vi "Topo & GridSpectr_DriftCorrection_zSpec_v16.vi"(6 "Internal use":string, 7 "Grid param":T1 {"height (m)" format="%#_6p"; "width (m)" format="%#_6p"; "center Y (m)" format="%#_6p"; "center X (m)" format="%#_6p"}, 8 "Error in (no error)":errorcluster, 9 "Points Y/Index Y":i32, 10 "Points X/Index X":i32, 11 "Method":enum16{"init", "run", "end"}(ring)=enum."end") -> (0 "Error out":errorcluster)   [LabVIEW 2014]
doc: "Example of a measurement VI to be used in the \"Experiments on a Grid\" tool as external VI.\n\nThis example measure the topography and spectroscopy data. The spectroscopy measurements are taken on a subgrid. The data are saved to a sxm and a binary file.\n\n- Nanonis Programming Interface -"
uses:
  <userlib>/Nanonis Prog Interface V5/Scan/Grid/GridPatternGet.vi
  <userlib>/Nanonis Prog Interface V5/Scan/Grid/LinePatternGet.vi
  <userlib>/Nanonis Prog Interface V5/Nanonis Prog Interface.lvlib
panel:
  in  "autoStop":bool
  in  "trigger 2 >Hz":sgl format="%#_6p"
  in  "trigger1 < Hz":sgl format="%#_6p"
  out "zFile":refnum<file>
  out "last z adjustment":sgl format="%#_6p"
  in  "during Spec Bias (V)":sgl format="%#_5p"
  in  "type":u16(ring)=1 items=["Line", "Grid"]
  in  "readjust setpoint every":i32=4
  in  "Correct Drift":bool=TRUE
  in  "Email when finished":string="cornelius.krull@monash.edu"
  in  "STS z offset":dbl format="%#_6p"
  out "ETA":timestamp
  out "remaining":dbl format="%<%H:%M:%S>t"
  out "Progress":u8(slide) scale=0.0..100.0 scale format="%#.1g"
  out "total Points":i32
  in  "preSTS delay [ms]":u32=500
  in  "ref Bias":dbl=0.02 format="%#_6p"
  in  "Imaging Bias":dbl=0.02 format="%#_6p"
  in  "max applied Drift Correction":i32=20 min=1 max=100 step=1 format="%.0p"
  in  "Correlate":u16(ring) items=["first Frame", "successive Frames"]
  out "Topo Images taken":i32=14
  in  "Increment":i32=40
  in  "Threshold":i32=2 min=1 step=1
  in  "tip Speed (m/s)":sgl=2e-09 format="%.2p"
  out "X drift":i32
  out "Y drift":i32
  out "Last Drift detected":i32=40
  in  "MaxImagesBack":i32=40
  in  "Channel index (0-23)":u8(ring) items=["Current"=0, "Z (m)"=14]
  in  "File name":string="symmetric_node"
  in  "ref Current":dbl=5e-12 format="%#_6p"
  in  "Imaging Current":dbl=5e-12 format="%#_6p"
  in  "zdrift \nDuration (s)":dbl
  in  "Correct z drift":bool
  out "Status":string="finishing"
  in  "Drift correction Pixels":i32=256 caption="Topo Pixels"
  out "Y Offset":dbl format="%#_6p"
  out "X Offset":dbl format="%#_6p"
  out "Points taken":dbl=14.0
  in  "Drift Correction every":i32=40
  # "z Spectroscopy"
  # "GRID points"
  # "Increase this if no Drift was detected for \na certain number of images"
  # "%"
  # "time (HH:MM:SS)"
  # "images back"
  # "% of image size"
  # "RUN smart tilt before starting the GRID\nImg Angle = 0\nmove tip to reference point for tip height"
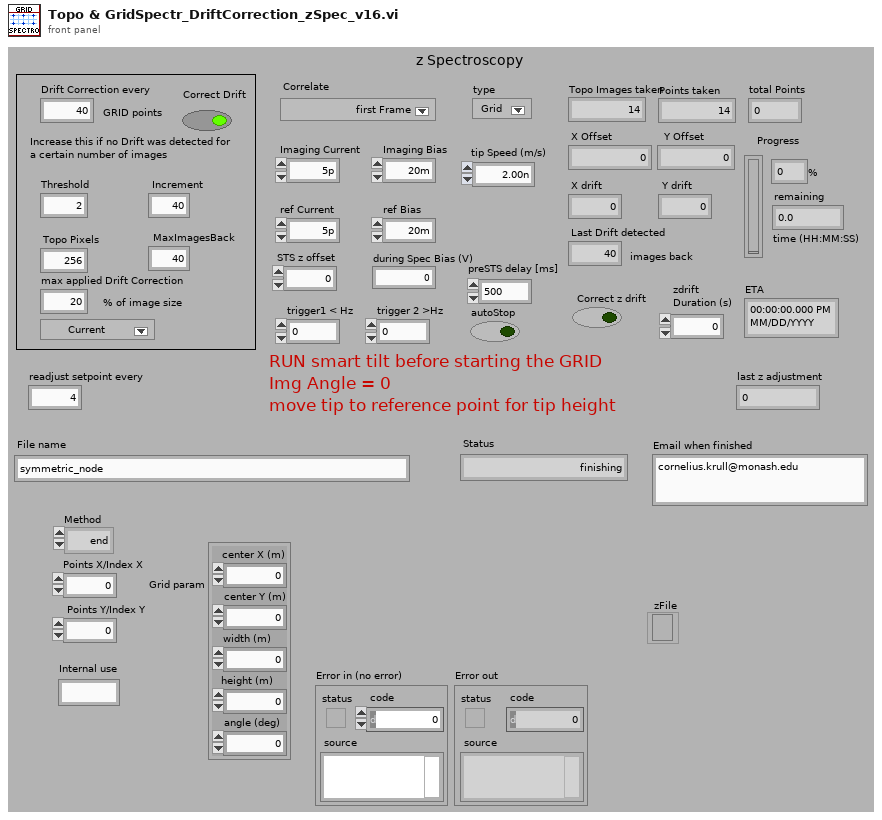
[diagram p1: front panel]
types:
  T1 = cluster{"center X (m)":sgl, "center Y (m)":sgl, "width (m)":sgl, "height (m)":sgl, "angle (deg)":sgl}
  T2 = enum16{"open", "replace", "create", "open or create", "replace or create", "replace or create with confirmation"}
  T3 = cluster{"Z averaging time (s)":sgl, "Z offset (m)":sgl, "Initial settling time (s)":sgl}
  T4 = cluster{"Drift correction Pixels":i32, "Imaging Current":dbl, "STS Current":dbl, "MaxImagesBack":i32, "tip Speed (m/s)":sgl, "Threshold":i32, "Increment":i32, "Correlate":u16, "max applied Drift Correction":i32, "Imaging Bias":dbl, "Move Current":dbl, "Move Bias":dbl, "STS Bias":dbl, "preSTS delay [ms]":u32, "STS z offset":dbl, "Correct Drift":bool, "Lockin ON/OFF":bool}
  T5 = cluster{"center X":sgl, "center Y":sgl, "angle":sgl, "width":sgl, "height":sgl, "# pixels":i32, "# lines":i32}
  T6 = cluster{"Name":string, "Calibration":sgl, "Offset":sgl, "Channel index":i32}[]
  T7 = cluster{"up/down":bool, "time/line":sgl, "start time":timestamp, "end time":timestamp}
  T8 = cluster{"Points X/Index X":i32, "Points Y/Index Y":i32}
  T9 = cluster{"Z averaging time (s)":sgl, "Initial settling time (s)":sgl}
  T10 = cluster{"Max. slew rate (m/s)":sgl, "Settling time (s)":sgl, "Integration time (s)":sgl}
  T11 = cluster{"End settling time (s)":sgl, "Z control time (s)":sgl}
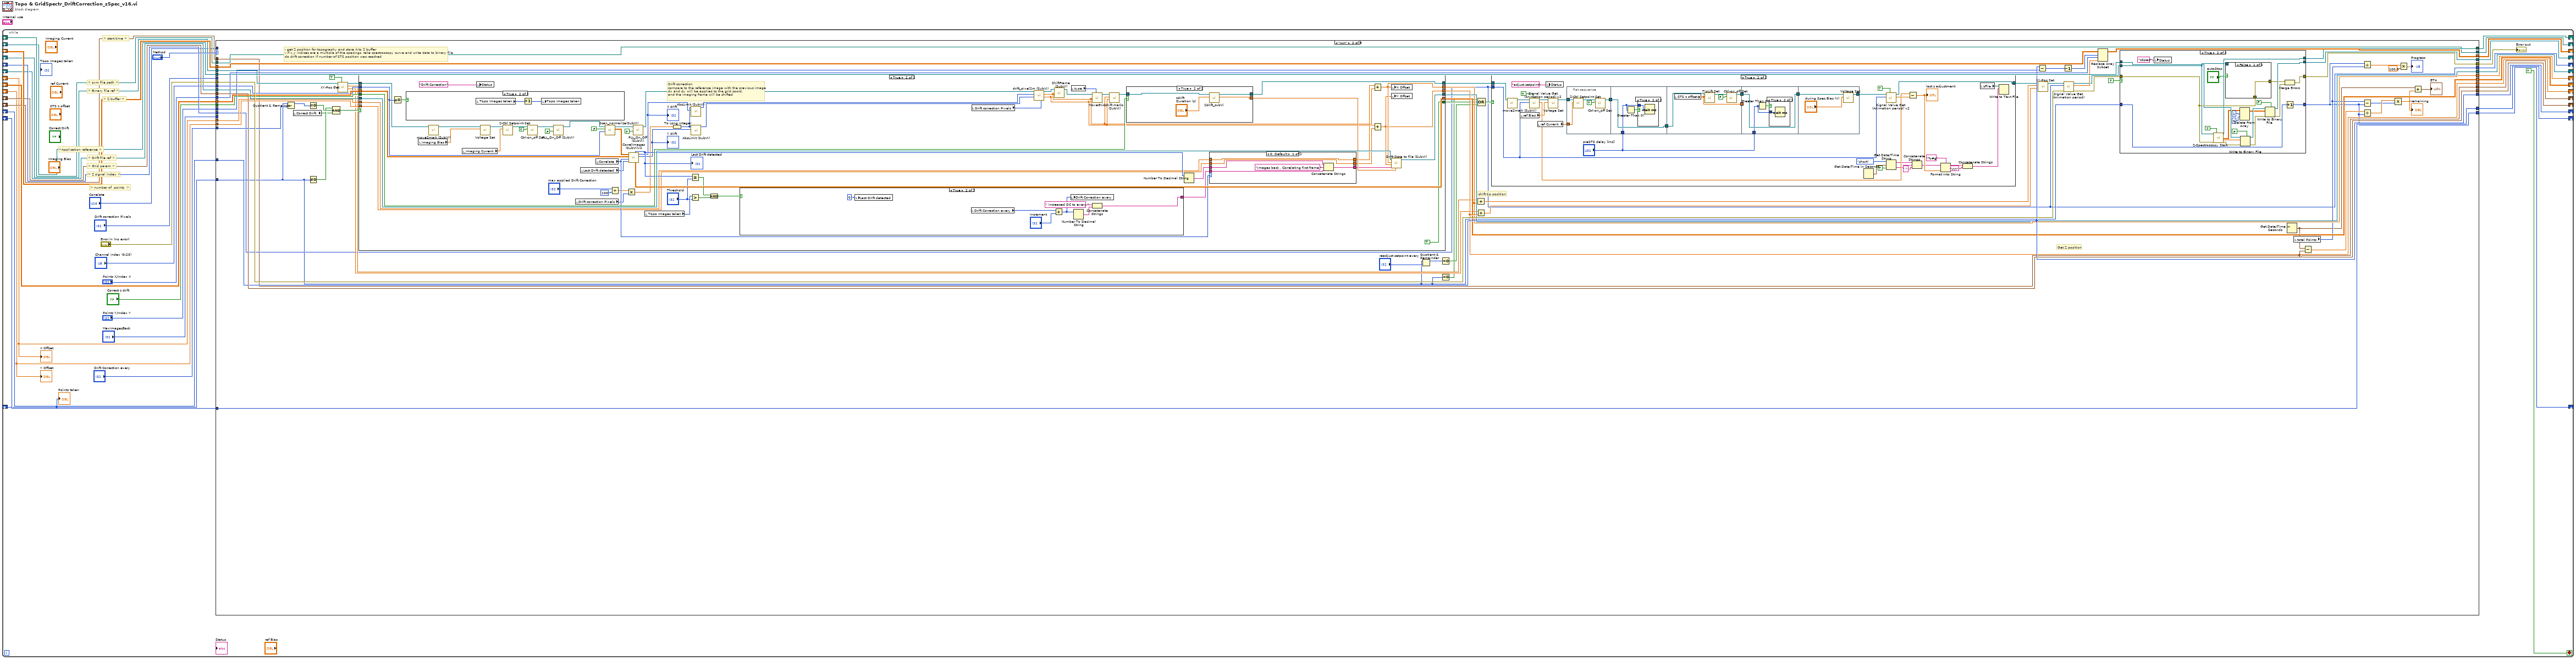
[diagram p0: block diagram]
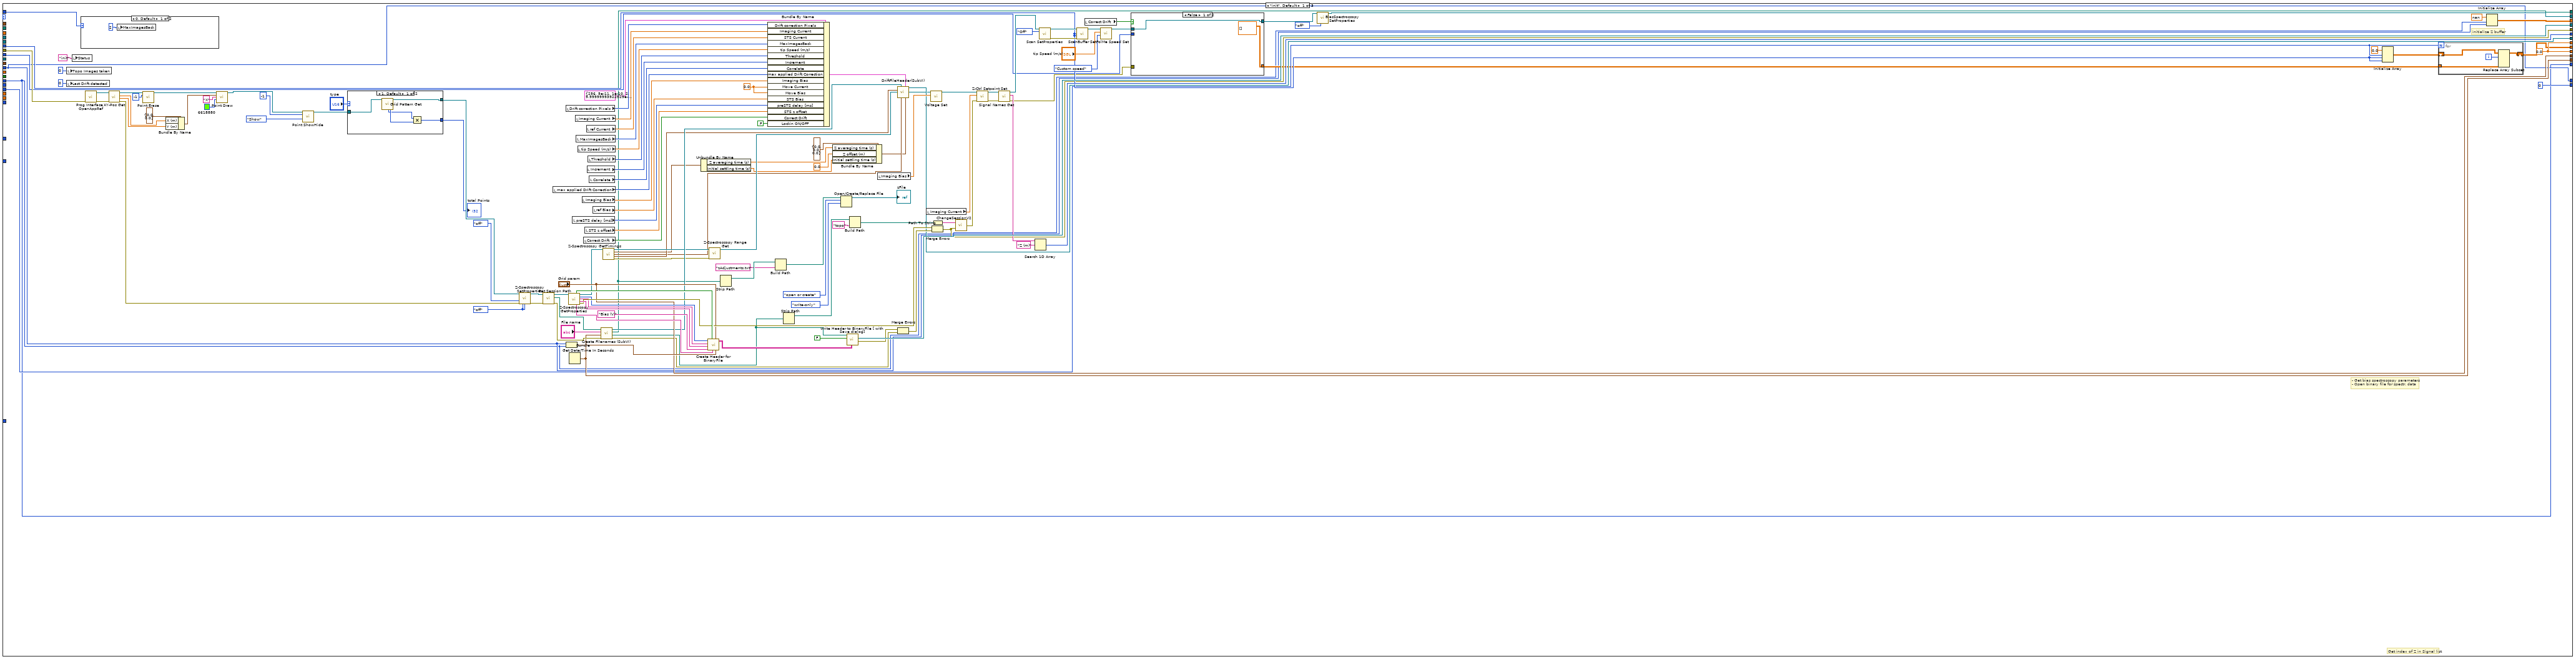
[diagram p2: hidden frame]
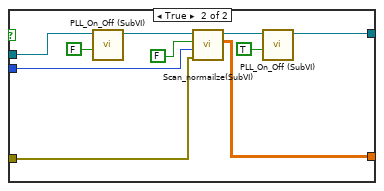
[diagram p3: hidden frame]
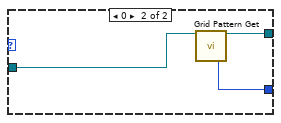
[diagram p4: hidden frame]
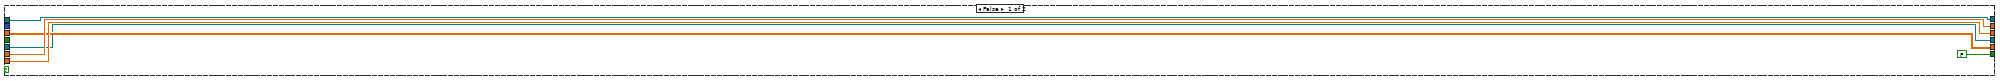
[diagram p9: hidden frame]
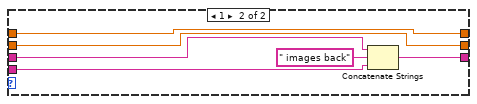
[diagram p10: hidden frame]
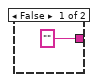
[diagram p12: hidden frame]
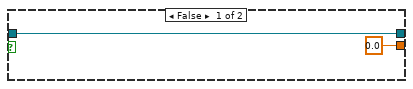
[diagram p13: hidden frame]
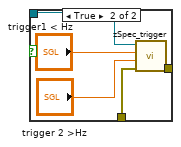
[diagram p15: hidden frame]
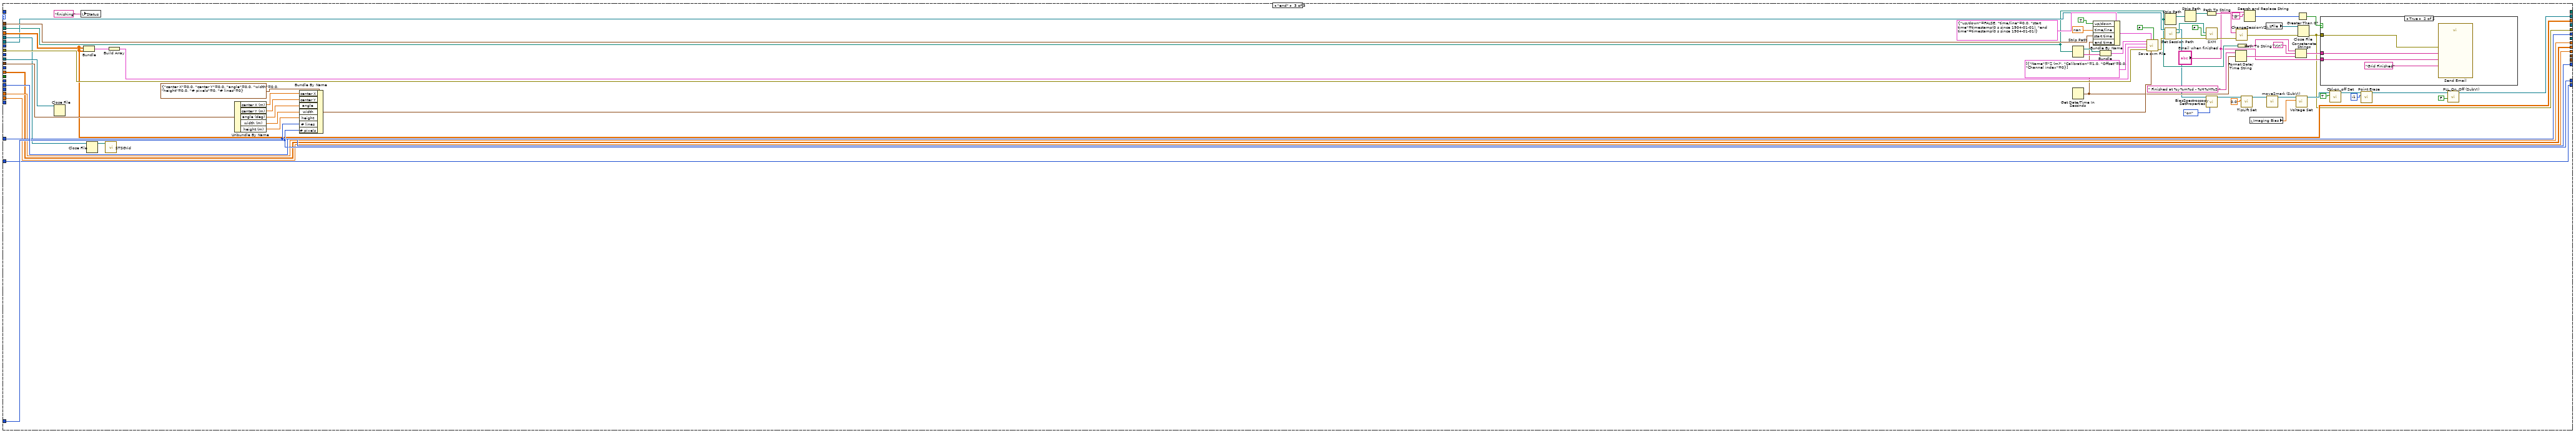
[diagram p16: hidden frame]
diagram:
  n1 = while {
    shift-right: [w21] -> _
    shift-left: _ -> [w38]
    shift-right: [w33] -> _
    shift-left: _ -> [w32]
    shift-right: [w30] -> _
    shift-left: _ -> [w31]
    shift-right: [w29] -> _
    shift-left: _ -> [w28]
    shift-right: [w27] -> _
    shift-left: _ -> [w26]
    shift-right: [w25] -> _
    shift-left: _ -> [w24]
    shift-right: [w23] -> _
    shift-left: _ -> [w22]
    shift-right: [w20] -> _
    shift-left: _ -> [w19]
    shift-right: [w18] -> _
    shift-left: _ -> [w17]
    shift-right: [w16] -> _
    shift-left: _ -> [w9]
    shift-right: [w15] -> _
    shift-left: _ -> [w8]
    shift-right: [w14] -> _
    shift-left: _ -> [w11]
    shift-right: [w13] -> _
    shift-left: _ -> [w10]
    shift-right: [w6] -> _
    shift-left: _ -> [w5]
    stop <- TRUE stop-if-true
    # "> Drift file ref >"
    # "> number of  points  >"
    # "> Grid param >"
    # "> start time >"
    # ">Application reference >"
    # "> Z signal index >"
    # "> Binary file ref >"
    # "> Z buffer >"
    # "> sxm file path >"
    n2 = case shown="\"run\"" "Method" {
      tunnel: [w49 w259 _] -> w21
      tunnel: w38 -> [_ w259 w470]
      tunnel: "Error in (no error)" -> [w143 w252 w500]
      tunnel: [w123 w258 w447] -> w36
      tunnel: "Points X/Index X" -> [w42 w253 _]
      tunnel: "Points Y/Index Y" -> [w41 w246 _]
      tunnel: [w169 w256 w489] -> w33
      tunnel: w32 -> [_ w257 w489]
      tunnel: w31 -> [_ w255 w482]
      tunnel: [w161 w254 _] -> w30
      tunnel: [w159 w196 w512] -> w29
      tunnel: w28 -> [_ w196 w512]
      tunnel: [w108 w239 w445] -> w27
      tunnel: w26 -> [_ w223 w475]
      tunnel: ["Grid param" w249 _] -> w25
      tunnel: w24 -> [_ w249 w499]
      tunnel: [w141 w214 _] -> w23
      tunnel: w22 -> [_ w214 w507]
      tunnel: [w41 w247 w490] -> w20
      tunnel: w19 -> [_ w247 w490]
      tunnel: [w42 w248 w491] -> w18
      tunnel: w17 -> [_ w248 w491]
      tunnel: [w152 w229 w488] -> w16
      tunnel: [w152 w234 w486] -> w15
      tunnel: [w137 w228 w483] -> w14
      tunnel: [0 w212 w487] -> w13
      tunnel: w10 -> [_ w198 w487]
      tunnel: "Drift Correction every" -> [_ w242 _]
      tunnel: w11 -> [_ w233 w483]
      tunnel: w9 -> [_ w240 w488]
      tunnel: w8 -> [_ w226 w486]
      tunnel: "Drift correction Pixels" -> [w136 _ _]
      tunnel: [w104 w231 _] -> w6
      tunnel: w5 -> [_ w232 w484]
      tunnel: "Correct z drift" -> [_ w230 _]
      tunnel: "Channel index (0-23)" -> [w86 w227 _]
      tunnel: "MaxImagesBack" -> [w135 _ _]
      tunnel: "Correlate" -> [w116 _ _]
      frame "init", Default {
        w51 = 0.0 ("Move Current")
        w106 = enum16{"no change", "on", "off"}."off" ("Save dialog")
        w152 = 0.0
        # "- Get bias spectroscopy parameters\n- Open binary file for spectr. data"
        # "initialize Z buffer"
        # "Get index of Z in Signal list"
        n3 = local write "Topo Images taken"(0 ("Images taken")) -> ()
        n4 = local write "Last Drift detected"(0 ("Last Drift detected")) -> ()
        n5 = local write "Status"("init" ("Status")) -> ()
        n6 = case shown="0, Default" w116 {
          frame 0, Default {
            n7 = local write "MaxImagesBack"(2 ("StepsBack")) -> ()
          }
          frame 1 {
          }
        }
        n8 = call <userlib>:"Prog Interface - OpenAppRef.vi"("Error in (no error)"=w143) -> ("Error out"=w81:errorcluster, "Application reference"=w83:refnum<vi>)  [unwired: 5 in]
        n9 = call <userlib>:"XY-Pos Get.vi"("error in (no error)"=w81, "Application ref in"=w83) -> ("error out"=w82:errorcluster, "Y (m)"=w75:sgl, "X (m)"=w76:sgl, "Application ref out"=w57:refnum<vi>)  [unwired: 5 in]
        n10 = call <userlib>:"Point Erase.vi"("Application ref in"=w57, "Point index (-1=All points)"=-1) -> ("Application ref out"=w56:refnum<vi>)  [unwired: 12 in, 1 out]
        n11 = Bundle By Name(cluster=cluster{"X (m)":sgl, "Y (m)":sgl} {"X (m)"=0.0, "Y (m)"=0.0} ("Point Coordinates"), "X (m)"=w76, "Y (m)"=w75) -> (w77:cluster{"X (m)":sgl, "Y (m)":sgl})
        n12 = call <userlib>:"Point Draw.vi"("Application ref in"=w56, "Point Coordinates"=w77, "Text"="X", "Color"=u32 6618880) -> ("Application ref out"=w61:refnum<vi>)  [unwired: 10 in, 1 out]
        n13 = call <userlib>:"Point ShowHide.vi"("Application ref in"=w61, "Point index (-1=All points)"=-1, "Show/Hide"=enum16{"Show", "Hide"}."Show") -> ("Application ref out"=w60:refnum<vi>)  [unwired: 11 in, 1 out]
        n14 = case shown="1, Default" "type" {
          tunnel: [w186 w189] -> w110
          tunnel: [w183 w187] -> w109
          tunnel: w60 -> [w182 w188]
          frame 1, Default {
            n15 = call-poly <userlib>:"Grid Pattern Get.vi"("Application ref in"=w182) -> ("Points Y"=w184:i32, "Points X"=w185:i32, "Application ref out"=w186:refnum<vi>)  [unwired: 10 in, 6 out]
            n16 = Multiply(x=w184, y=w185) -> (x*y=w183:i32)
          }
          frame 0 {
            n17 = call-poly <userlib>:"Grid Pattern Get.vi"("Application ref in"=w188) -> ("Points"=w187:i32, "Application ref out"=w189:refnum<vi>)  [unwired: 12 in, 5 out]
          }
        }
        "total Points" <- w109
        n18 = call <userlib>:"Z-Spectroscopy SetProperties.vi"("Application ref in"=w110, "Autosave"=enum16{"no change", "on", "off"}."off" ("Autosave (no change)"), "error in (no error)"=w82, "Save dialog"=w106, "Save all sweeps (no change)"=w106) -> ("Application ref out"=w119:refnum<vi>, "error out"=w118:errorcluster)  [unwired: 9 in]
        n19 = call <userlib>:"Get Session Path.vi"("error in (no error)"=w118, "Application ref in"=w119) -> ("error out"=w142:errorcluster, "Session path"=w129:path, "Application ref out"=w120:refnum<vi>)  [unwired: 7 in]
        n20 = local read "max applied Drift Correction"() -> (w92:i32)
        n21 = local read "Drift correction Pixels"() -> (w100:i32)
        n22 = Bundle("Points X/Index X"=w42, "Points Y/Index Y"=w41) -> (w164:T8)  [unwired: 1 in]
        n23 = call <userlib>:"Z-Spectroscopy GetProperties.vi"("Application ref in"=w120) -> ("Backward sweep"=w165:bool, "Application ref out"=w72:refnum<vi>, "Number of points"=w156:i32, "Channels"=w155:string[], "Parameters"=w163:string[], "Fixed parameters"=w158:string[], "error out"=w162:errorcluster)  [unwired: 7 in, 1 out]
        n24 = Get Date/Time In Seconds() -> (seconds since 1Jan1904=w141:timestamp)
        n25 = local read "preSTS delay [ms]"() -> (w89:u32)
        n26 = local read "Imaging Current"() -> (w99:dbl)
        n27 = local read "MaxImagesBack"() -> (w96:i32)
        n28 = local read "tip Speed (m/s)"() -> (w97:sgl)
        n29 = local read "Imaging Bias"() -> (w91:dbl)
        n30 = local read "Correct Drift"() -> (w87:bool)
        n31 = local read "STS z offset"() -> (w88:dbl)
        n32 = local read "ref Current"() -> (w98:dbl)
        n33 = local read "Increment"() -> (w94:i32)
        n34 = local read "Threshold"() -> (w95:i32)
        n35 = local read "Correlate"() -> (w93:u16)
        n36 = local read "ref Bias"() -> (w90:dbl)
        n37 = call "Create Filenames (SubVI).vi"("error in (no error)"=w142, "seconds since 1Jan1904"=w141, "File name"="File name", "Session path"=w129) -> ("error out"=w132:errorcluster, "binFilePath"=w125:path, "topoFilePath"=w49:path, "Drift File out"=w105:refnum<file>)  [unwired: 4 in]
        n38 = call <userlib>:"Z-Spectroscopy GetTimings.vi"("Application ref in"=w72) -> ("Application ref out"=w73:refnum<vi>, "Initialization"=w68:T9, "Sweep Timing"=w69:T10, "End of Sweep"=w70:T11, "Error out"=w74:errorcluster)  [unwired: 10 in]
        n39 = Unbundle By Name(w68) -> ("Z averaging time (s)"=w65:sgl, "Initial settling time (s)"=w64:sgl)
        n40 = call <userlib>:"Create Header for BinaryFile.vi"("Grid points"=w164, "Grid param"="Grid param", "Fixed parameters"=w158, "Backward sweep"=w165, "Sweep signal"="Bias (V)" ("Sweep Signal"), "Parameters"=w163, "Channels"=w155, "Points per sweep"=w156) -> ("Header (fixed attributes)"=w167:string[][])  [unwired: 3 in]
        n41 = call <userlib>:"Z-Spectroscopy Range Get.vi"("error in (no error)"=w74, "Application ref in"=w73) -> ("Application ref out"=w71:refnum<vi>)  [unwired: 5 in, 3 out]
        n42 = Strip Path(path=w49) -> (stripped path=w48:path)  [unwired: 1 out]
        n43 = Bundle By Name(cluster=T4 {"Drift correction Pixels"=256, "Imaging Current"=5e-11, "STS Current"=1e-10, "MaxImagesBack"=2, "tip Speed (m/s)"=1e-08, "Threshold"=2, "Increment"=64, "Correlate"=0, "max applied Drift Correction"=20, "Imaging Bias"=-0.02, "Move Current"=1.5e-11, "Move Bias"=-0.02, "STS Bias"=0.1, "preSTS delay [ms]"=1000, "STS z offset"=-1.7e-10, "Correct Drift"=TRUE, "Lockin ON/OFF"=TRUE} ("Drift Correction"), "Drift correction Pixels"=w100, "Imaging Current"=w99, "STS Current"=w98, "MaxImagesBack"=w96, "tip Speed (m/s)"=w97, "Threshold"=w95, "Increment"=w94, "Correlate"=w93, "max applied Drift Correction"=w92, "Imaging Bias"=w91, "Move Current"=w51, "Move Bias"=w51, "STS Bias"=w90, "preSTS delay [ms]"=w89, "STS z offset"=w88, "Correct Drift"=w87, "Lockin ON/OFF"=FALSE) -> (w102:T4)
        n44 = Build Path(base path=w48, name or relative path="zAdjustments.txt") -> (appended path=w46:path)
        n45 = Strip Path(path=w125) -> (stripped path=w128:path)  [unwired: 1 out]
        n46 = Bundle By Name(cluster=T3 {"Z averaging time (s)"=0.0, "Z offset (m)"=0.0, "Initial settling time (s)"=0.0} ("Initialization"), "Z averaging time (s)"=w65, "Z offset (m)"=sgl 0.0, "Initial settling time (s)"=w64) -> (w66:T3)
        n47 = Open/Create/Replace File(file path (use dialog)=w46, operation (0:open)=T2."open or create", access (0:read/write)=enum16{"read/write", "read-only", "write-only"}."write-only") -> (refnum out=→"zFile":refnum<file>)  [unwired: 3 in, 2 out]
        n48 = call <userlib>:"Write Header to BinaryFile [ with Save dialog].vi"("Fixed Attributes"=w167, "Show Dialog? (T)"=FALSE, "Filename"=w125) -> ("Error out"=w133:errorcluster, "File ref"=w161:refnum<file>)  [unwired: 5 in, 2 out]
        n49 = Build Path(base path=w128, name or relative path="topo") -> (appended path=w126:path)
        n50 = local read "Imaging Bias"() -> (w112:dbl)
        n51 = call "DriftFileHeader(SubVI).vi"("Byte Stream File in"=w105, "Drift Correction"=w102, "End of Sweep"=w70, "Application ref in"=w71, "Sweep Timing"=w69, "Initialization"=w66) -> ("Byte Stream File out"=w104:refnum<file>, "Application ref out"=w103:refnum<vi>)  [unwired: 8 in]
        n52 = Merge Errors(w133, w132) -> (w134:errorcluster)
        n53 = local read "Imaging Current"() -> (w111:dbl)
        n54 = call <userlib>:"Voltage Set.vi"("Bias (V)"=w112, "Application ref in"=w103) -> ("Application ref out"=w113:refnum<vi>)  [unwired: 8 in, 1 out]
        n55 = Path To String(path=w126) -> (string=w124:string)
        n56 = Merge Errors(w162, w134) -> (w123:errorcluster)
        n57 = call "ChangeSessionV2.vi"("error in (no error)"=w123, "Session"=w124) -> ("error out"=w122:errorcluster)
        n58 = call <userlib>:"Z-Ctrl Setpoint Set.vi"("error in (no error)"=w122, "Z Controller setpoint"=w111, "Application ref in"=w113) -> ("error out"=w144:errorcluster, "Application ref out"=w145:refnum<vi>)  [unwired: 7 in]
        n59 = call <userlib>:"Signal Names Get.vi"("error in (no error)"=w144, "Application ref in"=w145) -> ("error out"=w85:errorcluster, "Signals Names"=w157:string[], "Application ref out"=w148:refnum<vi>)  [unwired: 5 in]
        n60 = Search 1D Array(1D array=w157, element="Z (m)") -> (index of element=w159:i32)  [unwired: 1 in]
        n61 = call <userlib>:"Scan SetProperties.vi"("Application ref in"=w148, "Continuous scan"=enum16{"No change", "On", "Off"}."Off") -> ("Application ref out"=w150:refnum<vi>, "Error out"=w149:errorcluster)  [unwired: 12 in]
        n62 = call <userlib>:"ScanBuffer Set.vi"("Application ref in"=w150, "Pixels"=w136, "Lines"=w136, "error in (no error)"=w149) -> ("Application ref out"=w114:refnum<vi>)  [unwired: 10 in, 1 out]
        n63 = local read "Correct Drift"() -> (w52:bool)
        n64 = call <userlib>:"FolMe Speed Set.vi"("Speed Setting (Custom)"=enum32{"Scan speed", "Custom speed"}."Custom speed", "Speed (m/s)"="tip Speed (m/s)", "Application ref in"=w114) -> ("Application ref out"=w54:refnum<vi>)  [unwired: 5 in, 1 out]
        n65 = case shown="False" w52 {
          tunnel: w86 -> [_ w181]
          tunnel: w85 -> [_ w180]
          tunnel: [dbl[][] [] ("Array") w179] -> w84
          tunnel: w54 -> [w171 w177]
          tunnel: [w171 w172] -> w50
          frame False {
          }
          frame True {
            n66 = call "PLL_On_Off (SubVI).vi"("Output ON/OFF (F=OFF)"=FALSE, "Application in"=w177) -> ("Application out"=w176:refnum<vi>)  [unwired: 8 in, 1 out]
            n67 = call "Scan_normailze(SubVI).vi"("error in (no error)"=w180, "Channel index (0-23)"=w181, "Normalization"=FALSE ("Boolean"), "Application in"=w176) -> ("Array"=w179:dbl[][], "Application out"=w173:refnum<vi>)  [unwired: 5 in, 1 out]
            n68 = call "PLL_On_Off (SubVI).vi"("Output ON/OFF (F=OFF)"=TRUE, "Application in"=w173) -> ("Application out"=w172:refnum<vi>)  [unwired: 8 in, 1 out]
          }
        }
        n69 = call <userlib>:"BiasSpectroscopy SetProperties.vi"("Application ref in"=w50, "Z-Controller hold (no change)"=enum16{"no change", "on", "off"}."off") -> ("Application ref out"=w108:refnum<vi>)  [unwired: 12 in, 1 out]
        n70 = Initialize Array(0.0 ("element"), w135, w136, w136) -> (w138:dbl[][][])
        n71 = for {
          N: w135 -> [_]
          tunnel: w84 -> [w193]
          shift-right: [w192] -> w137
          shift-left: w138 -> [w194]
          i -> [w191]
          n72 = Replace Array Subset(array=w194, new element=w193, index (dim 0)=w191) -> (w192:dbl[][][])  [unwired: 2 in]
        }
        n73 = Initialize Array(sgl nan ("element"), w41, w42) -> (w169:sgl[][])
      }
      frame "run" {
        # "shift tip position"
        # "Get Z position"
        # "- get Z position for topography and store it to Z buffer\n- if x,y indices are a multiple of the spacings, take spectroscopy curve and write data to binary file\ndo drift correction if number of STS position was reached"
        n74 = Quotient & Remainder(x=w198, y=w242) -> (x-y*floor(x/y)=w243:i32)  [unwired: 1 out]
        n75 = local read "Correct Drift"() -> (w206:bool)
        n76 = Equal To 0?(x=w243) -> (x = 0?=w241:bool)
        n77 = Not Equal To 0?(x=w198) -> (x != 0?=w224:bool)
        n78 = Compound Arithmetic op=AND(w224, w241, w206) -> (w225:bool)
        n79 = call <userlib>:"XY-Pos Get.vi"("Wait for newest data (F=False)"=TRUE, "Application ref in"=w223) -> ("Y (m)"=w219:sgl, "X (m)"=w220:sgl, "Application ref out"=w222:refnum<vi>)  [unwired: 5 in, 1 out]
        n80 = case shown="True" w225 {
          tunnel: w222 -> [w320 w332]
          tunnel: [w320 w377] -> w203
          tunnel: w233 -> [w317 w373]
          tunnel: [w319 w375] -> w229
          tunnel: [w318 w374] -> w234
          tunnel: w240 -> [w319 w356]
          tunnel: w226 -> [w318 w354]
          tunnel: [w317 w369] -> w228
          tunnel: w232 -> [w316 w380]
          tunnel: [w316 w379] -> w231
          tunnel: w230 -> [_ w376]
          tunnel: w227 -> [_ w360]
          tunnel: [FALSE TRUE] -> w200
          frame False {
          }
          frame True {
            # "Drift correction \ncompare to the reference image with the previous image \ndx and dy will be applied to the grid coord, \nand the imaging frame will be shifted"
            n81 = Greater Or Equal To 0?(x=w360) -> (x >= 0?=w359:bool)
            n82 = case shown="True" w359 {
              frame False {
              }
              frame True {
                n83 = local read "Topo Images taken"() -> (w395:i32)
                n84 = Increment(x=w395) -> (x+1=w394:i32)
                n85 = local write "Topo Images taken"(w394) -> ()
              }
            }
            n86 = local read "Imaging Bias"() -> (w339:dbl)
            n87 = call "move2mark (SubVI).vi"("Application in"=w332) -> ("Application out"=w331:refnum<vi>)  [unwired: 10 in]
            n88 = local read "Imaging Current"() -> (w338:dbl)
            n89 = local write "Status"("Drift Correction" ("Status")) -> ()
            n90 = call <userlib>:"Voltage Set.vi"("Bias (V)"=w339, "Application ref in"=w331) -> ("Application ref out"=w340:refnum<vi>)  [unwired: 8 in, 1 out]
            n91 = call <userlib>:"Z-Ctrl Setpoint Set.vi"("Z Controller setpoint"=w338, "Application ref in"=w340) -> ("Application ref out"=w330:refnum<vi>)  [unwired: 8 in, 1 out]
            n92 = call <userlib>:"Ctrl-on_off Set.vi"("Z Controller ON/OFF"=TRUE, "Application ref in"=w330) -> ("Application ref out"=w328:refnum<vi>)  [unwired: 8 in, 1 out]
            n93 = call "PLL_On_Off (SubVI).vi"("Output ON/OFF (F=OFF)"=FALSE, "Application in"=w328) -> ("Application out"=w327:refnum<vi>)  [unwired: 8 in, 1 out]
            n94 = local read "Drift correction Pixels"() -> (w348:i32)
            n95 = local read "Last Drift detected"() -> (w351:i32)
            n96 = local read "Correlate"() -> (w357:u16)
            n97 = call "Scan_normailze(SubVI).vi"("Channel index (0-23)"=w360, "Normalization"=FALSE ("Boolean"), "Application in"=w327) -> ("Array"=w370:dbl[][], "Application out"=w325:refnum<vi>)  [unwired: 6 in, 1 out]
            n98 = Divide(x="max applied Drift Correction", y=100) -> (x/y=w347:dbl)
            n99 = Multiply(x=w347, y=w348) -> (x*y=w349:dbl)
            n100 = call "CorrelImages (SubVI)v2.vi"("last drift detected"=w351, "Correlate"=w357, "Ref Array"=w373, "New Image"=w370) -> ("Y drift"=w345:i32, "X drift"=w342:i32, "Ref Array out"=w369:dbl[][][], "Queue Steps"=w358:i32)  [unwired: 4 in]
            "X drift" <- w342
            "Y drift" <- w345
            "Last Drift detected" <- w358
            n101 = call "PLL_On_Off (SubVI).vi"("Output ON/OFF (F=OFF)"=TRUE, "Application in"=w325) -> ("Application out"=w322:refnum<vi>)  [unwired: 8 in, 1 out]
            n102 = local read "Topo Images taken"() -> (w362:i32)
            n103 = To Long Integer(number=w349) -> (32bit integer=w341:i32)
            n104 = Greater Or Equal?(x=w358, y="Threshold") -> (x >= y?=w364:bool)
            n105 = Greater?(x=w362, y="Threshold") -> (0:w361:bool)
            n106 = call "AbsLimit (SubVI).vi"("in"=w342, "Abslimt"=w341) -> ("Numeric out"=w344:i32)  [unwired: 9 in]
            n107 = call "AbsLimit (SubVI).vi"("in"=w345, "Abslimt"=w341) -> ("Numeric out"=w343:i32)  [unwired: 9 in]
            n108 = And(x=w364, y=w361) -> (x .and. y?=w363:bool)
            n109 = case shown="True" w363 {
              tunnel: ["" w399] -> w365
              frame False {
              }
              frame True {
                n110 = local write "Last Drift detected"(0 ("Last Drift detected")) -> ()
                n111 = local read "Drift Correction every"() -> (w398:i32)
                n112 = Add(x=w398, y="Increment") -> (x+y=w402:i32)
                n113 = local write "Drift Correction every"(w402) -> ()
                n114 = Number To Decimal String(number=w402) -> (decimal integer string=w401:string)  [unwired: 1 in]
                n115 = Concatenate Strings(" Increased DC to every " ("string"), w401) -> (w399:string)
              }
            }
            n116 = local read "Drift correction Pixels"() -> (w367:i32)
            n117 = call "drift_pixel2m (SubVI).vi"("Application in"=w322, "X drift"=w344, "Y drift"=w343, "Drift correction Pixels"=w367) -> ("Application out"=w366:refnum<vi>, "x drift"=w336:sgl, "y drift"=w335:sgl)  [unwired: 2 in, 1 out]
            n118 = call "ShiftFrame (SubVI).vi"("Y shift"=w335, "X shift"=w336, "Application in"=w366) -> ("Application out"=w368:refnum<vi>)  [unwired: 8 in]
            n119 = local read "type"() -> (w321:u16)
            n120 = call "MoveGrid.vi"("type"=w321, "y"=w335, "x"=w336, "Application ref in"=w368) -> ("Application ref out"=w334:refnum<vi>)  [unwired: 6 in, 1 out]
            n121 = call "shift marks (SubVI).vi"("y"=w335, "x"=w336, "Application in"=w334) -> ("Application out"=w333:refnum<vi>)  [unwired: 7 in, 1 out]
            n122 = case shown="True" w376 {
              tunnel: [0.0 ("z drift") w409] -> w378
              tunnel: w333 -> [w404 w408]
              tunnel: [w404 w407] -> w377
              frame False {
              }
              frame True {
                n123 = call "Zdrift_subVi.vi"("Duration"="zdrift \nDuration (s)", "Application in"=w408) -> ("z drift"=w409:dbl, "Application out"=w407:refnum<vi>)  [unwired: 7 in, 1 out]
              }
            }
            n124 = Number To Decimal String(number=w358) -> (decimal integer string=w372:string)  [unwired: 1 in]
            n125 = case shown="0, Default" w357 {
              tunnel: w372 -> [w382 w393]
              tunnel: [w387 w392] -> w371
              tunnel: w365 -> [w385 w390]
              tunnel: w356 -> [w383 w389]
              tunnel: [w383 w389] -> w355
              tunnel: w354 -> [w384 w388]
              tunnel: [w384 w388] -> w353
              frame 0, Default {
                n126 = Concatenate Strings(w382, "images back , Correlating first frame " ("string"), w385) -> (w387:string)
              }
              frame 1 {
                n127 = Concatenate Strings(w393, " images back" ("string"), w390) -> (w392:string)
              }
            }
            n128 = Add(x=w355, y=w336) -> (x+y=w375:dbl)
            n129 = Add(x=w335, y=w353) -> (x+y=w374:dbl)
            n130 = local write "X Offset"(w375) -> ()
            n131 = local write "Y Offset"(w374) -> ()
            n132 = call "Drift Data to file (SubVI).vi"("z drift"=w378, "Comment"=w371, "y Drift"=w374, "X drift"=w375, "Byte Stream File in"=w380) -> ("Byte Stream File out"=w379:refnum<file>)  [unwired: 6 in]
          }
        }
        n133 = Quotient & Remainder(x=w198, y="readjust setpoint every") -> (x-y*floor(x/y)=w199:i32)  [unwired: 1 out]
        n134 = Equal To 0?(x=w199) -> (x = 0?=w202:bool)
        n135 = Equal To 0?(x=w198) -> (x = 0?=w197:bool)
        n136 = Add(x=w220, y=w229) -> (x+y=w236:dbl)
        n137 = Add(x=w219, y=w234) -> (x+y=w235:dbl)
        n138 = Compound Arithmetic op=OR(w197, w200, w202) -> (w201:bool)
        n139 = case shown="True" w201 {
          tunnel: [w260 w277] -> w204
          tunnel: w203 -> [w260 w293]
          tunnel: w196 -> [_ w279]
          frame False {
          }
          frame True {
            n140 = call "move2mark (SubVI).vi"("Application in"=w293) -> ("Application out"=w282:refnum<vi>)  [unwired: 10 in]
            n141 = local read "ref Bias"() -> (w292:dbl)
            n142 = call <userlib>:"Signal Value Get (Animation period) v2.vi"("Wait for newest data (F=False)"=TRUE, "Signal index (0-79)"=w279, "Application ref in"=w282) -> ("Signal value"=w275:sgl, "Application ref out"=w281:refnum<vi>)  [unwired: 5 in, 1 out]
            n143 = local read "ref Current"() -> (w289:dbl)
            n144 = local write "Status"("adjust setpoint" ("Status")) -> ()
            n145 = call <userlib>:"Voltage Set.vi"("Bias (V)"=w292, "Application ref in"=w281) -> ("Application ref out"=w290:refnum<vi>)  [unwired: 8 in, 1 out]
            n146 = flat-sequence {
              tunnel: w290 -> [w298]
              tunnel: [w295] -> w288
              tunnel: w289 -> [w297]
              tunnel: w288 -> [w301]
              tunnel: [w301] -> w287
              tunnel: "preSTS delay [ms]" -> [w299]
              tunnel: w287 -> [w306]
              tunnel: [w303] -> w291
              tunnel: [w304] -> w285
              tunnel: w291 -> [w310]
              tunnel: "preSTS delay [ms]" -> [w309]
              tunnel: w285 -> [_]
              tunnel: [w310] -> w283
              tunnel: [w312] -> w278
              tunnel: w283 -> [w313]
              frame #0 {
                n147 = call <userlib>:"Z-Ctrl Setpoint Set.vi"("Z Controller setpoint"=w297, "Application ref in"=w298) -> ("Application ref out"=w296:refnum<vi>)  [unwired: 8 in, 1 out]
                n148 = call <userlib>:"Ctrl-on_off Set.vi"("Z Controller ON/OFF"=TRUE, "Application ref in"=w296) -> ("Application ref out"=w295:refnum<vi>)  [unwired: 8 in, 1 out]
              }
              frame #1 {
                n149 = Greater Than 0?(x=w299) -> (x > 0?=w300:bool)
                n150 = case shown="True" w300 {
                  tunnel: w299 -> [_ w302]
                  frame False {
                  }
                  frame True {
                    n151 = Wait (ms)(milliseconds to wait=w302) -> ()  [unwired: 1 out]
                  }
                }
              }
              frame #2 {
                n152 = local read "STS z offset"() -> (w304:dbl)
                n153 = call <userlib>:"TipLift Set.vi"("TipLift (m)"=w304, "Application ref in"=w306) -> ("Application ref out"=w305:refnum<vi>)  [unwired: 8 in, 1 out]
                n154 = call <userlib>:"Ctrl-on_off Set.vi"("Z Controller ON/OFF"=FALSE, "Application ref in"=w305) -> ("Application ref out"=w303:refnum<vi>)  [unwired: 8 in, 1 out]
              }
              frame #3 {
                n155 = Greater Than 0?(x=w309) -> (x > 0?=w308:bool)
                n156 = case shown="True" w308 {
                  tunnel: w309 -> [_ w311]
                  frame False {
                  }
                  frame True {
                    n157 = Wait (ms)(milliseconds to wait=w311) -> ()  [unwired: 1 out]
                  }
                }
              }
              frame #4 {
                n158 = call <userlib>:"Voltage Set.vi"("Bias (V)"="during Spec Bias (V)", "Application ref in"=w313) -> ("Application ref out"=w312:refnum<vi>)  [unwired: 8 in, 1 out]
              }
            }
            n159 = Get Date/Time In Seconds() -> (seconds since 1Jan1904=w266:timestamp)
            n160 = call <userlib>:"Signal Value Get (Animation period) v2.vi"("Wait for newest data (F=False)"=TRUE, "Signal index (0-79)"=w279, "Application ref in"=w278) -> ("Signal value"=w274:sgl, "Application ref out"=w277:refnum<vi>)  [unwired: 5 in, 1 out]
            n161 = Get Date/Time String(date format (0)=enum16{"short", "long", "abbreviated"}."short", seconds (now)=w266, want seconds? (F)=TRUE) -> (date string=w270:string, time string=w269:string)
            n162 = Subtract(x=w275, y=w274) -> (x-y=w272:sgl)
            "last z adjustment" <- w272
            n163 = Concatenate Strings(w270, w269, "," ("string")) -> (w268:string)
            n164 = Format Into String(format string="%#g", initial string=w268, w272) -> (resulting string=w263:string)  [unwired: 1 in, 1 out]
            n165 = Concatenate Strings(w263, "\r\n") -> (w262:string)
            n166 = local read "zFile"() -> (w273:refnum<file>)
            n167 = Write to Text File(file (use dialog)=w273, text=w262) -> ()  [unwired: 2 in, 3 out]
          }
        }
        n168 = Subtract(x=w247, y=w246) -> (x-y=w245:i32)
        n169 = call <userlib>:"XY-Pos Set.vi"("Y (m)"=w235, "X (m)"=w236, "Application ref in"=w204) -> ("Application ref out"=w237:refnum<vi>)  [unwired: 5 in, 1 out]
        n170 = Decrement(x=w245) -> (x-1=w244:i32)
        n171 = call <userlib>:"Signal Value Get (Animation period).vi"("error in (no error)"=w252, "Signal index (0-47)"=w196, "Application ref in"=w237) -> ("error out"=w251:errorcluster, "Signal value"=w250:sgl, "Application ref out"=w238:refnum<vi>)  [unwired: 5 in]
        n172 = Replace Array Subset(array=w257, new element=w250, index (row)=w244, index (col)=w253) -> (w256:sgl[][])
        n173 = case shown="True" TRUE {
          tunnel: [w412 w415] -> w258
          tunnel: w255 -> [w413 w436]
          tunnel: [w413 w434] -> w254
          tunnel: w251 -> [w412 w418]
          tunnel: w238 -> [w411 w419]
          tunnel: [w411 w420] -> w239
          tunnel: [w410 w422] -> w212
          tunnel: w198 -> [w410 w423]
          frame False {
            # "Point indices aren't multiple of subgrid spacing\n=> no spectroscopy at this point"
          }
          frame True {
            n174 = local write "Status"("zSpec" ("Status")) -> ()
            n175 = call <userlib>:"Z-Spectroscopy Start.vi"("Application ref in"=w419, "Get data (F=False)"=TRUE ("Get Data (F)"), "error in (no error)"=w418) -> ("Application ref out"=w420:refnum<vi>, "Data"=w433:sgl[][], "Parameters"=w432:sgl[], "error out"=w425:errorcluster)  [unwired: 8 in, 1 out]
            n176 = case shown="False" "autoStop" {
              tunnel: w419 -> [_ w442]
              tunnel: w418 -> [w437 w439]
              tunnel: [w437 w438] -> w417
              frame False {
              }
              frame True {
                n177 = call "zSpec_trigger.vi"("Error in (no error)"=w439, "trigger 2"="trigger 2 >Hz", "trigger1"="trigger1 < Hz", "Application ref in"=w442) -> ("Error out"=w438:errorcluster)  [unwired: 5 in, 1 out]
              }
            }
            n178 = Delete From Array(array=w433, length=1, index (row)=0 ("index")) -> (array with subset deleted=w431:sgl[][])  [unwired: 1 in, 1 out]
            n179 = Write to Binary File(file (use dialog)=w436, data=w432, error in=w425, 5:FALSE ("prepend array or string size? (T)")) -> (refnum out=w435:refnum<file>, error out=w424:errorcluster)  [unwired: 2 in, 1 out]
            n180 = Write to Binary File(file (use dialog)=w435, data=w431, error in=w424, 5:FALSE ("prepend array or string size? (T)")) -> (refnum out=w434:refnum<file>, error out=w416:errorcluster)  [unwired: 2 in, 1 out]
            n181 = Merge Errors(w417, w416) -> (w415:errorcluster)
            n182 = Increment(x=w423) -> (x+1=w422:i32)
          }
        }
        n183 = Get Date/Time In Seconds() -> (seconds since 1Jan1904=w209:timestamp)
        n184 = local read "total Points"() -> (w215:i32)
        n185 = Subtract(x=w209, y=w214) -> (x-y=w213:dbl)
        n186 = Divide(x=w212, y=w215) -> (x/y=w218:dbl)
        n187 = Subtract(x=w215, y=w212) -> (x-y=w210:i32)
        n188 = Divide(x=w213, y=w212) -> (x/y=w211:dbl)
        n189 = Multiply(x=w211, y=w210) -> (x*y=w208:dbl)
        "remaining" <- w208
        n190 = Multiply(x=w218, y=100.0) -> (x*y=→"Progress":dbl)
        n191 = Add(x=w209, y=w208) -> (x+y=→"ETA":timestamp)
      }
      frame "end" {
        n192 = Close File(refnum=w484) -> ()  [unwired: 1 in, 2 out]
        n193 = local write "Status"("finishing" ("Status")) -> ()
        n194 = Bundle(w489, w489) -> (w511:cluster{sgl[][], sgl[][]})  [unwired: 1 in]
        n195 = Close File(refnum=w482) -> (path=w481:path)  [unwired: 1 in, 1 out]
        n196 = call "STSGrid.vi"("Binary Spectroscopy File"=w481) -> ()  [unwired: 11 in]
        n197 = Build Array(w511) -> (w510:cluster{sgl[][], sgl[][]}[])
        n198 = Unbundle By Name(w499) -> ("center X (m)"=w497:sgl, "center Y (m)"=w496:sgl, "angle (deg)"=w495:sgl, "width (m)"=w494:sgl, "height (m)"=w493:sgl)
        n199 = Bundle By Name(cluster=T5 {"center X"=0.0, "center Y"=0.0, "angle"=0.0, "width"=0.0, "height"=0.0, "# pixels"=0, "# lines"=0} ("Scanfield"), "center X"=w497, "center Y"=w496, "angle"=w495, "width"=w494, "height"=w493, "# lines"=w490, "# pixels"=w491) -> (w492:T5)
        n200 = Strip Path(path=w470) -> (stripped path=w503:path, name=w502:string)
        n201 = Get Date/Time In Seconds() -> (seconds since 1Jan1904=w466:timestamp)
        n202 = Bundle By Name(cluster=T7 {"up/down"=FALSE, "time/line"=0.0, "start time"=timestamp(0 s since 1904-01-01), "end time"=timestamp(0 s since 1904-01-01)} ("Scan param"), "up/down"=TRUE, "time/line"=sgl nan ("input 7"), "start time"=w507, "end time"=w466) -> (w506:T7)
        n203 = Bundle("stripped path"=w503, "name"=w502) -> (w501:cluster{"stripped path":path, "name":string})  [unwired: 1 in]
        n204 = call <userlib>:"Save sxm File.vi"("Auto file naming? (T)"=FALSE, "Scanfield"=w492, "Scan param"=w506, "error in (no error)"=w500, "Channels data"=w510, "Channels config"=T6 [{"Name"="Z (m)", "Calibration"=1.0, "Offset"=0.0, "Channel index"=0}], "Filename control"=w501) -> ("error out"=w476:errorcluster)  [unwired: 2 in, 2 out]
        n205 = Strip Path(path=w470) -> (stripped path=w480:path)  [unwired: 1 out]
        n206 = call <userlib>:"Get Session Path.vi"("error in (no error)"=w476, "Application ref in"=w475) -> ("error out"=w472:errorcluster, "Session path"=w474:path, "Application ref out"=w459:refnum<vi>)  [unwired: 7 in]
        n207 = Strip Path(path=w480) -> (stripped path=w479:path)  [unwired: 1 out]
        n208 = Path To String(path=w479) -> (string=w477:string)
        n209 = call "SXM.vi"("Path"=w474, "Delete"=FALSE, "error in"=w472) -> ("error out"=w471:errorcluster)  [unwired: 7 in]
        n210 = call <userlib>:"BiasSpectroscopy SetProperties.vi"("Application ref in"=w459, "Z-Controller hold (no change)"=enum16{"no change", "on", "off"}."on") -> ("Application ref out"=w457:refnum<vi>)  [unwired: 12 in, 1 out]
        n211 = Format Date/Time String(time format string (%c)=" Finished at %y%m%d - %H%M%S ", seconds (now)=w466) -> (date/time string=w465:string)  [unwired: 1 in]
        n212 = call "ChangeSessionV2.vi"("error in (no error)"=w471, "Session"=w477) -> ("error out"=w448:errorcluster)
        n213 = Path To String(path=w470) -> (string=w469:string)
        n214 = call <userlib>:"TipLift Set.vi"("TipLift (m)"=sgl 0.0, "Application ref in"=w457) -> ("Application ref out"=w454:refnum<vi>)  [unwired: 8 in, 1 out]
        n215 = Search and Replace String(input string="Email when finished", search string="@") -> (number of replacements=w461:i32)  [unwired: 6 in, 3 out]
        n216 = local read "Imaging Bias"() -> (w449:dbl)
        n217 = local read "zFile"() -> (w446:refnum<file>)
        n218 = call "move2mark (SubVI).vi"("Application in"=w454) -> ("Application out"=w450:refnum<vi>)  [unwired: 10 in]
        n219 = Concatenate Strings(w469, "\r\n", w465) -> (w468:string)
        n220 = call <userlib>:"Voltage Set.vi"("Bias (V)"=w449, "Application ref in"=w450) -> ("Application ref out"=w451:refnum<vi>)  [unwired: 8 in, 1 out]
        n221 = Greater Than 0?(x=w461) -> (x > 0?=w460:bool)
        n222 = Close File(refnum=w446, error in=w448) -> (error out=w447:errorcluster)  [unwired: 1 out]
        n223 = case shown="True" w460 {
          tunnel: w447 -> [_ w516]
          tunnel: w468 -> [_ w514]
          tunnel: "Email when finished" -> [_ w513]
          frame False {
          }
          frame True {
            n224 = call "Send Email"("error in"=w516, "Message"=w514, "Subject"="Grid Finished", "Recipients"=w513) -> ()  [unwired: 7 in, 1 out]
          }
        }
        n225 = call <userlib>:"Ctrl-on_off Set.vi"("Z Controller ON/OFF"=TRUE, "Application ref in"=w451) -> ("Application ref out"=w453:refnum<vi>)  [unwired: 8 in, 1 out]
        n226 = call <userlib>:"Point Erase.vi"("Application ref in"=w453, "Point index (-1=All points)"=-1) -> ("Application ref out"=w444:refnum<vi>)  [unwired: 12 in, 1 out]
        n227 = call "PLL_On_Off (SubVI).vi"("Output ON/OFF (F=OFF)"=FALSE, "Application in"=w444) -> ("Application out"=w445:refnum<vi>)  [unwired: 8 in, 1 out]
      }
    }
    "Error out" <- w36
    "Points taken" <- w10
    "X Offset" <- w9
    "Y Offset" <- w8
  }
